vi "Arrays 0.vi"() -> ()   [LabVIEW 2014]
panel:
  out "Array":i32[](array[numeric])
  in  "Max":i32
  in  "No. of elements":i32
  # "Arrays- Generate Array"
  # "Range"
  # "Array"
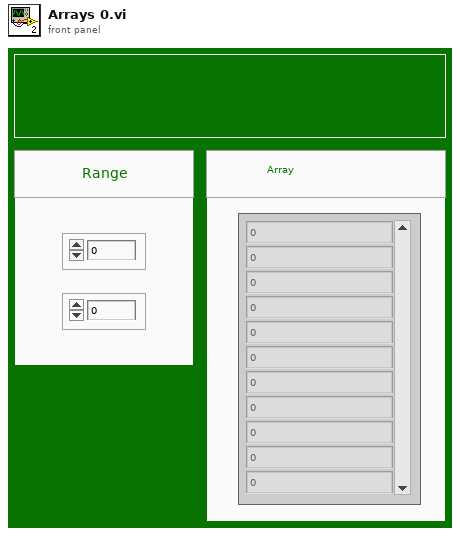
[diagram p1: front panel]
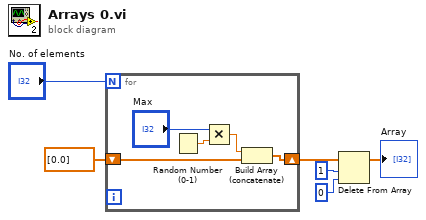
[diagram p0: block diagram]
diagram:
  n1 = for {
    N: "No. of elements" -> [_]
    shift-right: [w8] -> w6
    shift-left: dbl[] [0.0] -> [w7]
    n2 = Random Number (0-1)() -> (number: 0 to 1=w10:dbl)
    n3 = Multiply(x="Max", y=w10) -> (x*y=w9:dbl)
    n4 = Build Array (concatenate)(w9, w7) -> (w8:dbl[])
  }
  n5 = Delete From Array(array=w6, length=1, index=0) -> (array with subset deleted=→"Array":dbl[])  [unwired: 1 out]
